vi "WILT Agilent Setup.vi"(4 "Custom Agilent List":bool, 6 "Agilent Channel Assignment":path=path "C:/Work/Agilent Channel Assignment - Wilt.ini", 7 "Agilent Semaphore":T3[](array[typedef]), 8 "error in (no error)":errorcluster, 10 "Agilent Refs":refnum<visa-resource-name>[](array[refnum])=["AGILENT1", "AGILENT2", "AGILENT3", "AGILENT4", "AGILENT5", "AGILENT6", "AGILENT7"], 11 "File Locations":T1[](array[typedef])) -> (0 "error out":errorcluster, 3 "Data Out Array":T5, 5 "Agilent Switches":T4[](array[typedef]))   [LabVIEW 2016]
uses:
  Type Definitions/WILT Agilent Data Cluster.ctl
  Type Definitions/WILT Agilent Channel Definition.ctl
  Utility/Save File/File Setup (Public)/Type Definition/Save File DOE File Path Control.ctl
  Utility/Save File/File Setup (Public)/Type Definition/Save File DOE Data Save Filepaths.ctl
  Utility/Save File/File Setup.lvlib
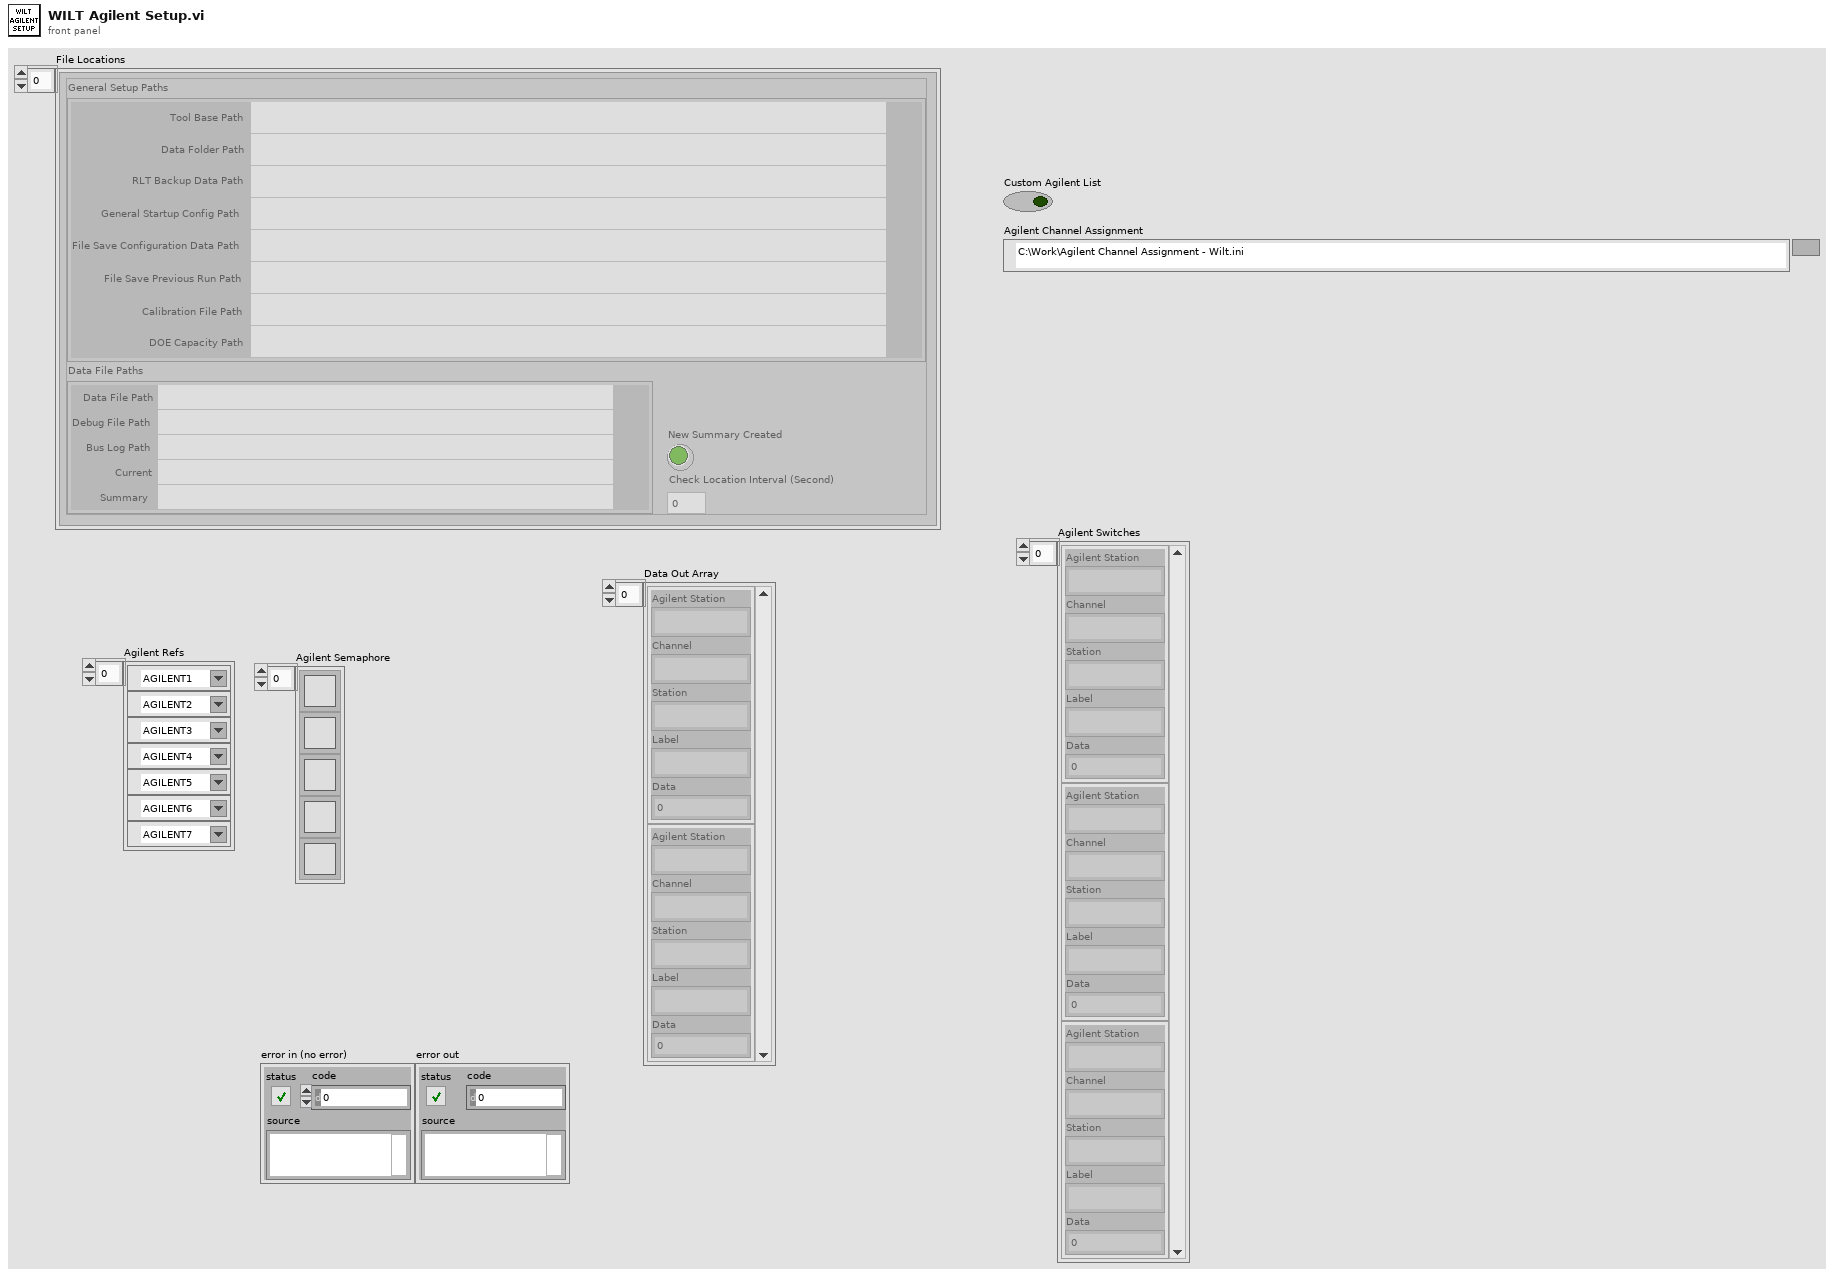
[diagram p1: front panel]
types:
  T1 = typedef "File Setup.lvlib/Save File DOE File Path Control.ctl" = cluster{"General Setup Paths":cluster{"Calibration File Path":path, "DOE Capacity Path":path, "Data Folder Path":path, "RLT Backup Data Path":path, "Tool Base Path":path, "General Startup Config Path":path, "File Save Previous Run Path":path, "File Save Configuration Data Path":path}, "Data File Paths":T2, "New Summary Created":bool, "Check Location Interval (Second)":i32}
  T2 = typedef "File Setup.lvlib/Save File DOE Data Save Filepaths.ctl" = cluster{"Data File Path":path, "Debug File Path":path, "Bus Log Path":path, "Current":path, "Summary":path}
  T3 = typedef "Semaphore RefNum" = refnum<k1>
  T4 = typedef "WILT Agilent Channel Definition.ctl" = cluster{"Channel":string, "Station":string, "Label":string, "Agilent Station":string, "Data":dbl}
  T5 = typedef "WILT Agilent Data Cluster.ctl" = T4[]
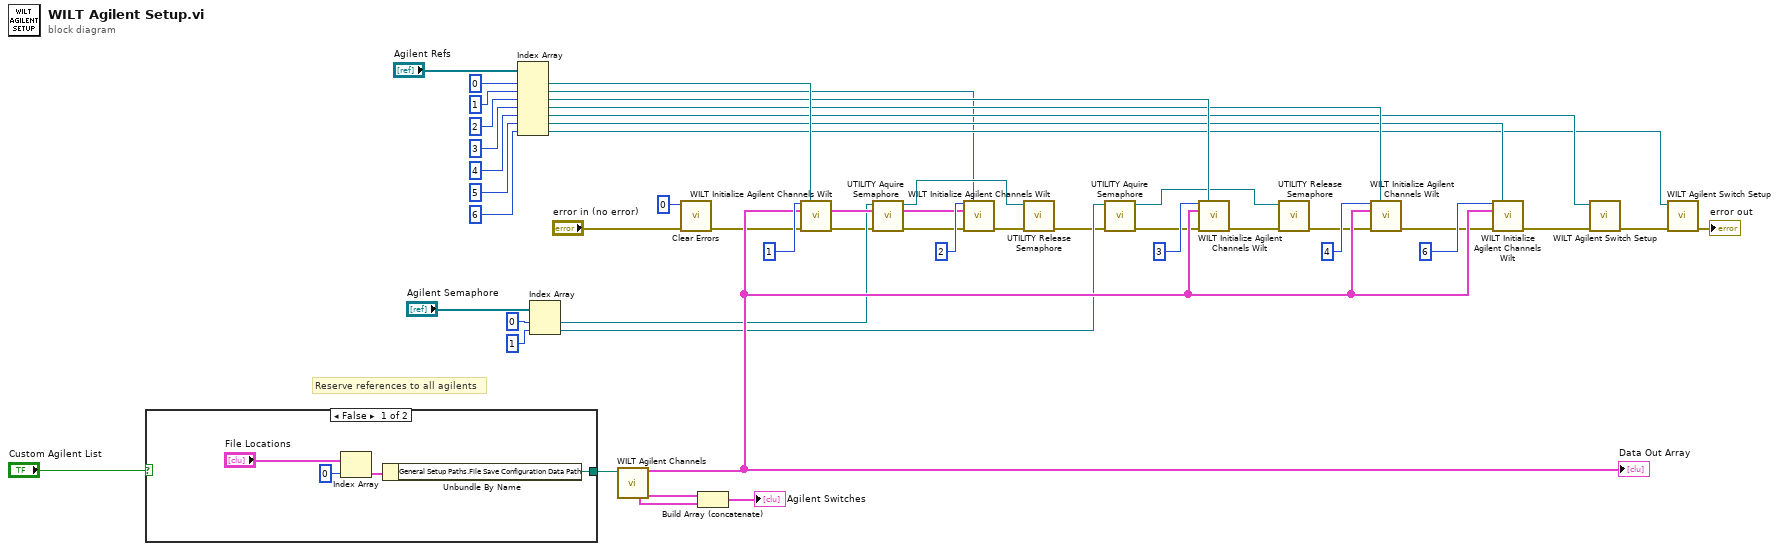
[diagram p0: block diagram]
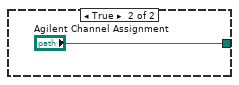
[diagram p2: hidden frame]
diagram:
  # "Reserve references to all agilents"
  n1 = case shown="False" "Custom Agilent List" {
    tunnel: [w48 "Agilent Channel Assignment"] -> w3
    frame False {
      n2 = Index Array(array="File Locations", index=0) -> (element=w49:T1)
      n3 = Unbundle By Name(w49) -> ("General Setup Paths.File Save Configuration Data Path"=w48:path)
    }
    frame True {
    }
  }
  n4 = Index Array(array="Agilent Refs", index #1=0 ("index"), index #2=1 ("index"), index #3=2 ("index"), index #4=3 ("index"), index #5=4 ("index"), index #6=5 ("index"), index #7=6 ("index")) -> (element #1=w39:refnum<visa-resource-name>, element #2=w2:refnum<visa-resource-name>, element #3=w36:refnum<visa-resource-name>, element #4=w34:refnum<visa-resource-name>, element #5=w21:refnum<visa-resource-name>, element #6=w26:refnum<visa-resource-name>, element #7=w20:refnum<visa-resource-name>)
  n5 = Index Array(array="Agilent Semaphore", index #1=0 ("index"), index #2=1 ("index")) -> (element #1=w16:T3, element #2=w15:T3)
  n6 = call "WILT Agilent Channels.vi"("file path (dialog if empty)"=w3) -> ("Data Out Array"=w31:T5, "Start Buttons"=w46:T4[], "Agilent Channel Water Valves"=w47:T4[])  [unwired: 9 in, 3 out]
  "Data Out Array" <- w31
  n7 = call <vilib>:"Clear Errors.vi"("error in (no error)"="error in (no error)", "specific error code to clear (0: all)"=0) -> ("error out"=w29:errorcluster)  [unwired: 4 in, 1 out]
  n8 = Build Array (concatenate)(w47, w46) -> (→"Agilent Switches":T4[])
  n9 = call "WILT Initialize Agilent Channels Wilt.vi"("Agilent Number"=1, "VISA Resource Name"=w39, "Data Array"=w31, "error in (no error)"=w29) -> ("error out"=w12:errorcluster)  [unwired: 10 in, 1 out]
  n10 = call "UTILITY Aquire Semaphore.vi"("error in (no error)"=w12, "Refnum in"=w16) -> ("error out"=w11:errorcluster, "Refnum out"=w14:T3)  [unwired: 7 in, 1 out]
  n11 = call "WILT Initialize Agilent Channels Wilt.vi"("Agilent Number"=2, "VISA Resource Name"=w2, "Data Array"=w31, "error in (no error)"=w11) -> ("error out"=w10:errorcluster)  [unwired: 10 in, 1 out]
  n12 = call "UTILITY Release Semaphore.vi"("error in (no error)"=w10, "Refnum in"=w14) -> ("error out"=w9:errorcluster)  [unwired: 9 in]
  n13 = call "UTILITY Aquire Semaphore.vi"("error in (no error)"=w9, "Refnum in"=w15) -> ("error out"=w8:errorcluster, "Refnum out"=w13:T3)  [unwired: 7 in, 1 out]
  n14 = call "WILT Initialize Agilent Channels Wilt.vi"("Agilent Number"=3, "VISA Resource Name"=w36, "Data Array"=w31, "error in (no error)"=w8) -> ("error out"=w7:errorcluster)  [unwired: 10 in, 1 out]
  n15 = call "UTILITY Release Semaphore.vi"("error in (no error)"=w7, "Refnum in"=w13) -> ("error out"=w6:errorcluster)  [unwired: 9 in]
  n16 = call "WILT Initialize Agilent Channels Wilt.vi"("Agilent Number"=4, "VISA Resource Name"=w34, "Data Array"=w31, "error in (no error)"=w6) -> ("error out"=w30:errorcluster)  [unwired: 10 in, 1 out]
  n17 = call "WILT Initialize Agilent Channels Wilt.vi"("Agilent Number"=6, "VISA Resource Name"=w26, "Data Array"=w31, "error in (no error)"=w30) -> ("error out"=w23:errorcluster)  [unwired: 10 in, 1 out]
  n18 = call "WILT Agilent Switch Setup.vi"("Error In"=w23, "VISA Resource Name"=w21) -> ("Error Out"=w22:errorcluster)  [unwired: 9 in]
  n19 = call "WILT Agilent Switch Setup.vi"("Error In"=w22, "VISA Resource Name"=w20) -> ("Error Out"=→"error out":errorcluster)  [unwired: 9 in]
